vi "ReversedEngineering_AttributeToDataType.vi"(1 "ClassInfo":cluster{"ClassNamn":string, "ClassPath":path}[](array[cluster]), 2 "Array":string[](array[string])) -> (0 "Attributes":T1[](array[typedef]))   [LabVIEW 2012]
uses:
  <resource>/Framework/Providers/Open_GDS/ClassProviders/Common/CommonVIs/CommonVIs_AttributeType.ctl
  <resource>/Framework/Providers/Open_GDS/ClassProviders/Common/CommonVIs/CommonVIs_AttributeDataType.ctl
  <resource>/Framework/Providers/Open_GDS/ClassProviders/Common/String/GDSString_AccessScopeModifierType.ctl
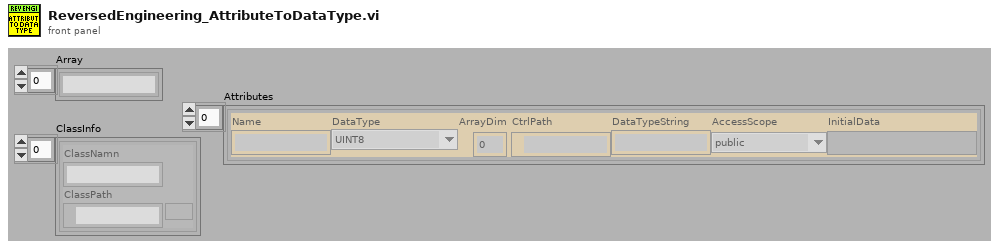
[diagram p1: front panel]
types:
  T1 = typedef "CommonVIs_AttributeType.ctl" = cluster{"Name":string, "DataType":T2, "ArrayDim":i32, "CtrlPath":path, "DataTypeString":string, "AccessScope":T3, "InitialData":variant}
  T2 = typedef "CommonVIs_AttributeDataType.ctl" = enum16{"UINT8", "INT8", "UINT16", "INT16", "UINT32", "INT32", "UINT64", "INT64", "SGL", "DBL", "EXT", "CSG", "CDB", "CXT", "TimeStamp", "STRING", "PATH", "BOOL", "ENUM", "RefNum", "VIRefNum", "LabVIEW Class", "Cluster", "Variant", "TypeDef", "Waveform", "LabVIEW Object", "Other", "void"}
  T3 = typedef "GDSString_AccessScopeModifierType.ctl" = enum16{"public", "private", "protected", "internal"}
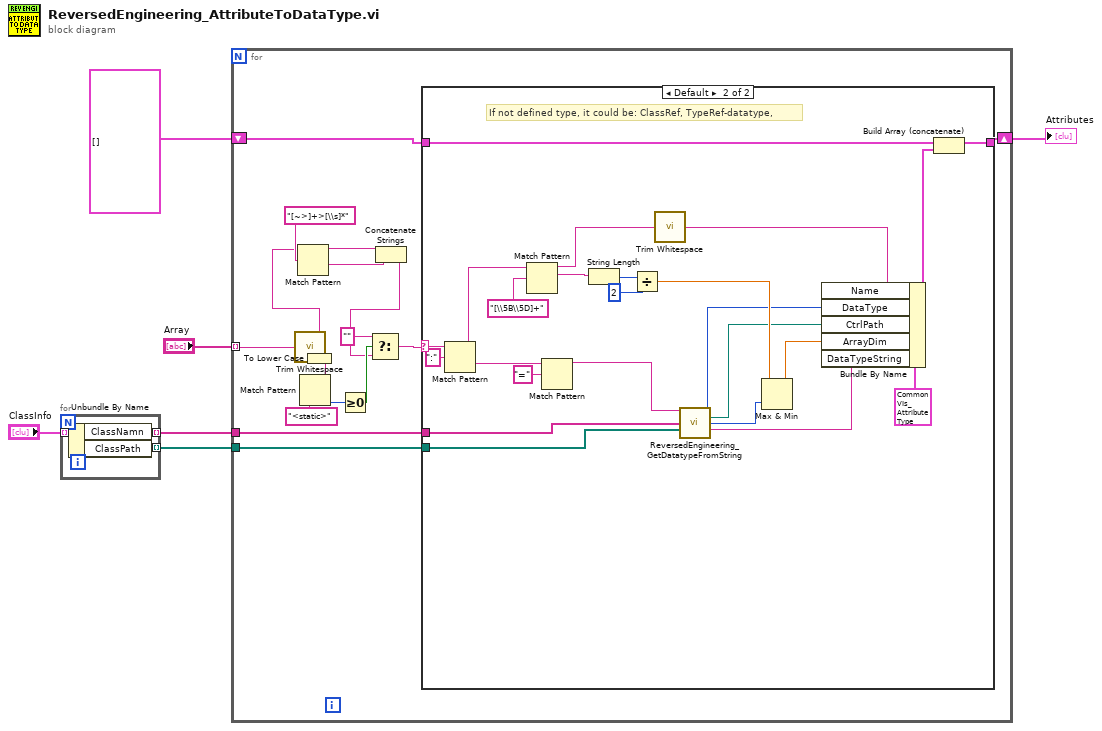
[diagram p0: block diagram]
diagram:
  n1 = for {
    tunnel: "ClassInfo" -> [w9] mode=indexing
    tunnel: [w8] -> w1 mode=indexing
    tunnel: [w7] -> w6 mode=indexing
    n2 = Unbundle By Name(w9) -> ("ClassNamn"=w8:string, "ClassPath"=w7:path)
  }
  n3 = for {
    tunnel: "Array" -> [w25] mode=indexing
    shift-right: [w23] -> w4
    shift-left: T1[] [] ("Attributes") -> [w24]
    tunnel: w1 -> [w22]
    tunnel: w6 -> [w21]
    n4 = call <vilib>:"Trim Whitespace.vi"("string"=w25) -> ("trimmed string"=w17:string)  [unwired: 1 in]
    n5 = Match Pattern(string=w17, regular expression="[~>]+>[\\s]*") -> (before substring=w20:string, after substring=w19:string)  [unwired: 3 out]
    n6 = To Lower Case(string=w17) -> (all lower case string=w15:string)
    n7 = Match Pattern(string=w15, regular expression="<static>") -> (offset past match=w14:i32)  [unwired: 4 out]
    n8 = Greater Or Equal To 0?(x=w14) -> (x >= 0?=w13:bool)
    n9 = Concatenate Strings(w20, w19) -> (w12:string)
    n10 = Select(t="", s=w13, f=w12) -> (s? t:f=w10:string)
    n11 = case shown="Default" w10 {
      selector: w10 -> [_ w47]
      tunnel: w24 -> [w26 w50]
      tunnel: [w26 w49] -> w23
      tunnel: w22 -> [_ w41]
      tunnel: w21 -> [_ w40]
      frame "" {
      }
      frame Default {
        # "If not defined type, it could be: ClassRef, TypeRef-datatype,"
        n12 = Match Pattern(string=w47, regular expression=":") -> (before substring=w39:string, after substring=w43:string)  [unwired: 3 out]
        n13 = Match Pattern(string=w39, regular expression="[\\5B\\5D]+") -> (before substring=w38:string, match substring=w34:string)  [unwired: 3 out]
        n14 = Match Pattern(string=w43, regular expression="=") -> (before substring=w42:string)  [unwired: 4 out]
        n15 = String Length(string=w34) -> (length=w35:i32)
        n16 = Divide(x=w35, y=2) -> (x/y=w33:dbl)
        n17 = call <vilib>:"Trim Whitespace.vi"("string"=w38) -> ("trimmed string"=w45:string)  [unwired: 1 in]
        n18 = call <resource>:"ReversedEngineering_GetDatatypeFromString.vi"("String"=w42, "ClassNames"=w41, "ClassPaths"=w40) -> ("AttributeDataType"=w29:T2, "ClassPath"=w28:path, "ArrayDimensions"=w32:i32, "DataTypeAsString(Array,default values removed)"=w30:string)  [unwired: 8 in, 1 out]
        n19 = Max & Min(x=w33, y=w32) -> (max(x,y)=w31:dbl)  [unwired: 1 out]
        n20 = Bundle By Name(cluster=T1 {"Name"="", "DataType"=enum."UINT8", "ArrayDim"=0, "CtrlPath"=path "", "DataTypeString"="", "AccessScope"=enum."public", "InitialData"=variant}, "Name"=w45, "DataType"=w29, "CtrlPath"=w28, "ArrayDim"=w31, "DataTypeString"=w30) -> (w27:T1)
        n21 = Build Array (concatenate)(w50, w27) -> (w49:T1[])
      }
    }
  }
  "Attributes" <- w4
